vi "Get SLSC Module Resource from Chassis IP.vi"(8 "error in (no error)":errorcluster, 10 "Slot Number":i32, 11 "Chassis Name or IP":string) -> (0 "error out":errorcluster, 3 "SLSC Device":refnum<k21>)   [LabVIEW 2020, in "VeriStand SLSC Scripting.lvlib"]
uses:
  VeriStand SLSC Scripting.lvlib
  <vilib>/nisyscfg/Close (System).vi
  <vilib>/SLSC/Initialize Session with Devices.vi
  <vilib>/SLSC/Close Session.vi
  <vilib>/nisyscfg/nisyscfg.lvlib
  <resource>/objmgr/nisysapi.rc
  <vilib>/SLSC/SLSC.lvlib
  <resource>/objmgr/slsc.rc
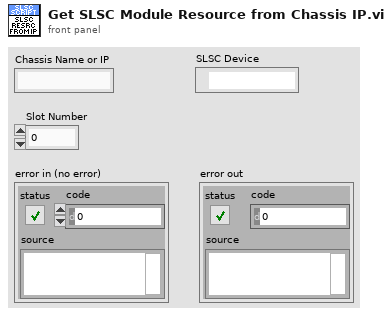
[diagram p1: front panel]
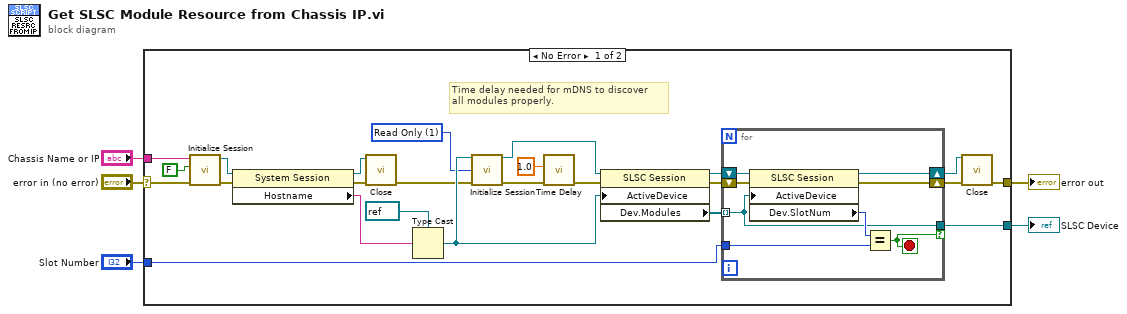
[diagram p0: block diagram]
diagram:
  n1 = case shown="No Error" "error in (no error)" {
    selector: "error in (no error)" -> [w26 w38]
    tunnel: "Chassis Name or IP" -> [w29 _]
    tunnel: [w25 w38] -> w3
    tunnel: [w22 _] -> w2
    tunnel: "Slot Number" -> [w21 _]
    frame No Error {
      w14 = 1 items=["None"=0, "Read Only"=1, "Read/Write"=3] ("reservation access (Read/Write)")
      # "Time delay needed for mDNS to discover\nall modules properly."
      n2 = call <vilib>:"Initialize Session.vi"("error in (no error)"=w26, "Force Property Refresh (T)"=FALSE, "Target (localhost)"=w29) -> ("error out"=w10:errorcluster, "Session out"=w9:refnum<k21>)  [unwired: 7 in]
      n3 = property class="System Session"(reference=w9, error in=w10) -> (reference out=w13:refnum<k21>, error out=w11:errorcluster, "Hostname"=w27:string)
      n4 = call-poly <vilib>:"Close.vi"("error in (no error)"=w11, "Session in"=w13) -> ("error out"=w15:errorcluster)  [unwired: 9 in]
      n5 = Type Cast(type=refnum<k21> refnum ("devices"), x=w27) -> (*(type *) &x=w18:refnum<k21>)
      n6 = call-poly <vilib>:"Initialize Session.vi"("devices"=w18, "reservation access (Read/Write)"=w14, "error in (no error)"=w15) -> ("session out"=w16:refnum<k21>, "error out"=w7:errorcluster)  [unwired: 11 in]
      n7 = call "Time Delay"("error in (no error)"=w7, "Delay Time (s)"=1.0) -> ("error out"=w6:errorcluster)  [unwired: 9 in]
      n8 = property class="SLSC Session"(reference=w16, error in=w6, "ActiveDevice"=w18) -> (reference out=w19:refnum<k21>, error out=w20:errorcluster, "Dev.Modules"=w28:refnum<k21>[])
      n9 = for {
        tunnel: w28 -> [w30] mode=indexing
        shift-right: [w35] -> w24
        shift-left: w20 -> [w36]
        shift-right: [w34] -> w23
        shift-left: w19 -> [w37]
        tunnel: w21 -> [w32]
        tunnel: [w30] -> w22 if=w31
        stop <- w31 stop-if-true
        n10 = property class="SLSC Session"(reference=w37, error in=w36, "ActiveDevice"=w30) -> (reference out=w34:refnum<k21>, error out=w35:errorcluster, "Dev.SlotNum"=w33:u32)
        n11 = Equal?(x=w33, y=w32) -> (x = y?=w31:bool)
      }
      n12 = call-poly <vilib>:"Close.vi"("session in"=w23, "error in (no error)"=w24) -> ("error out"=w25:errorcluster)  [unwired: 13 in]
    }
    frame Error {
    }
  }
  "error out" <- w3
  "SLSC Device" <- w2
